vi "Read DataGridView.vi"(8 "error in (no error)":errorcluster, 11 "Data Grid in":refnum<class "Data Grid.lvclass">) -> (0 "error out":errorcluster, 2 "DataGrid.lvlib:DataGridView.lvclass":refnum<class "DataGridView.lvclass">, 3 "Data Grid out":refnum<class "Data Grid.lvclass">)   [LabVIEW 2013, in "Table Manager.lvlib" / "Data Grid.lvclass"]
uses:
  Data Grid.lvclass
  <vilib>/LabVIEW DataGridView/source/DataGridView/DataGridView.lvclass
  Data Grid.lvclass/Data Grid.ctl
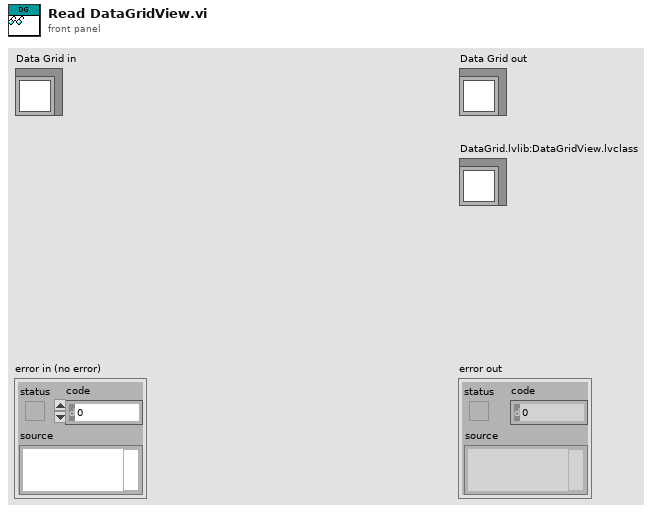
[diagram p1: front panel]
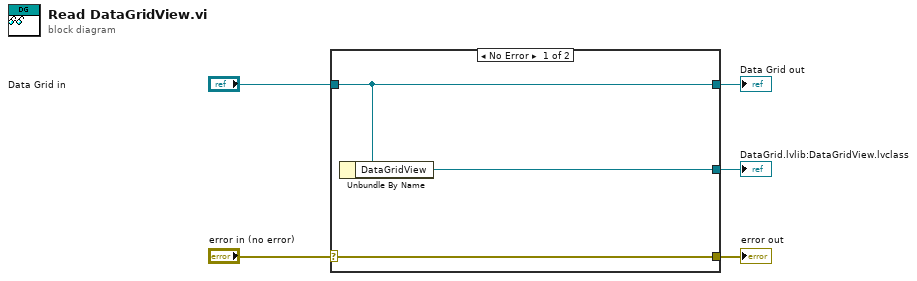
[diagram p0: block diagram]
diagram:
  n1 = case shown="No Error" "error in (no error)" {
    selector: "error in (no error)" -> [w8 w9]
    tunnel: [w8 w9] -> w4
    tunnel: [w7 w10] -> w2
    tunnel: "Data Grid in" -> [w7 w10]
    tunnel: [w6 _] -> w1
    frame No Error {
      n2 = Unbundle By Name(w7) -> ("DataGridView"=w6:refnum<class "DataGridView.lvclass">)
    }
    frame Error {
    }
  }
  "error out" <- w4
  "Data Grid out" <- w2
  "DataGrid.lvlib:DataGridView.lvclass" <- w1
